vi "trafficlight_main.vi"() -> ()   [LabVIEW 2022 SP3]
panel:
  in  "Stop":bool
  in  "Standby":bool
  out "TrafficLight":cluster{"red":bool, "orange":bool, "green":bool}
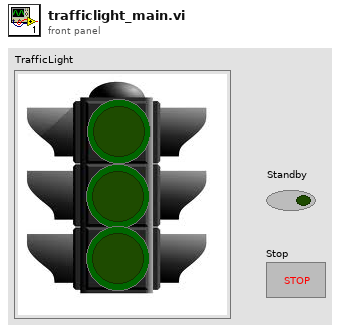
[diagram p1: front panel]
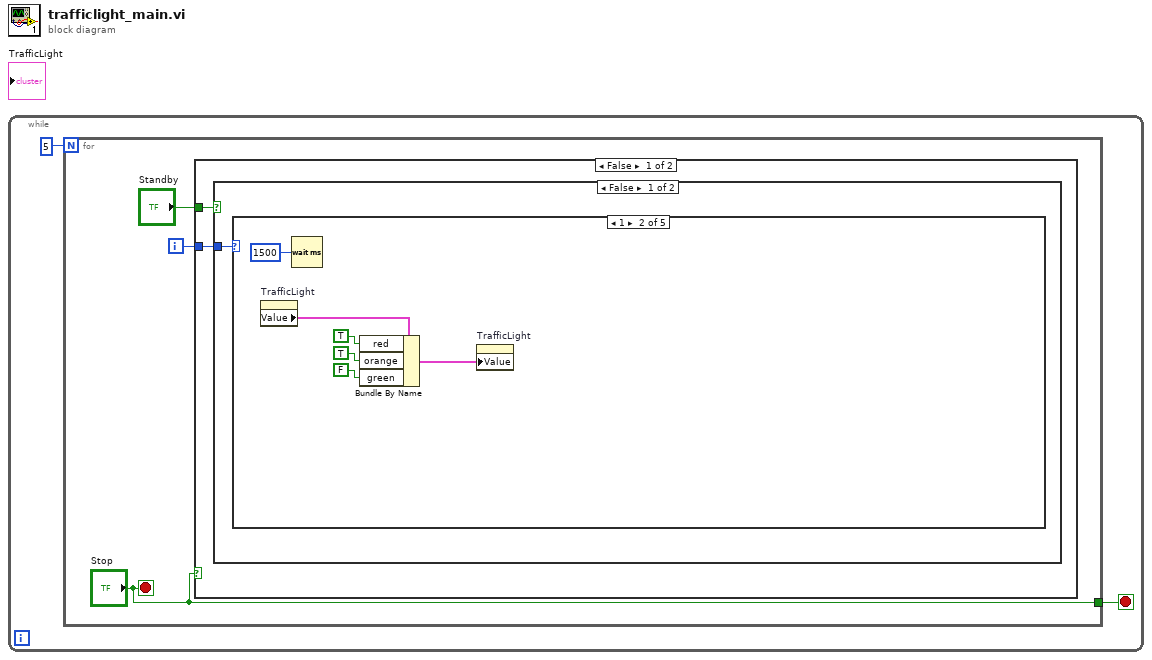
[diagram p0: block diagram]
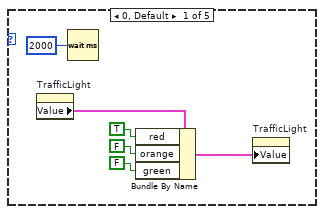
[diagram p2: hidden frame]
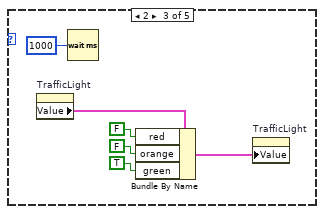
[diagram p3: hidden frame]
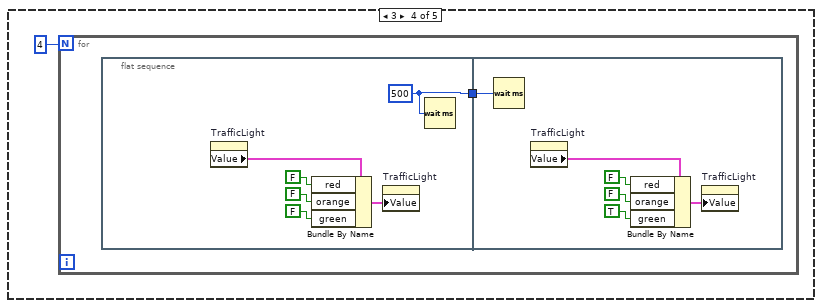
[diagram p4: hidden frame]
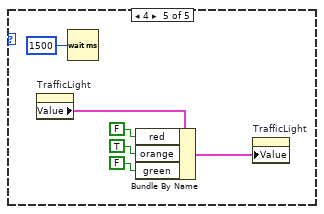
[diagram p5: hidden frame]
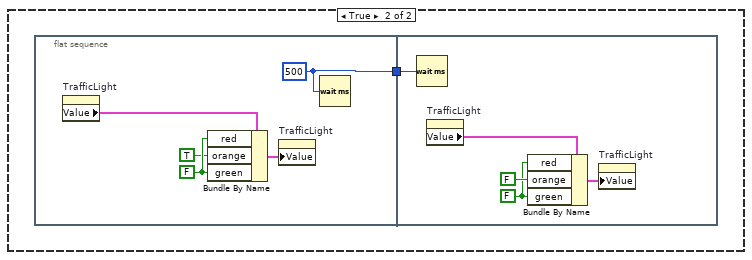
[diagram p6: hidden frame]
diagram:
  n1 = while {
    stop <- w1 stop-if-true
    n2 = for {
      N: 5 -> [_]
      tunnel: ["Stop"] -> w1
      i -> [w5]
      stop <- "Stop" stop-if-true
      n3 = case shown="False" "Stop" {
        tunnel: w5 -> [w7 _]
        tunnel: "Standby" -> [w6 _]
        frame False {
          n4 = case shown="False" w6 {
            tunnel: w7 -> [w8 _]
            frame False {
              n5 = case shown="1" w8 {
                frame 0, Default {
                  n6 = property on="TrafficLight" class="Clust (strict)"() -> ("Value"=w13:cluster{"red":bool, "orange":bool, "green":bool})  [unwired: 2 in, 2 out]
                  n7 = Wait (ms)(milliseconds to wait=u32 2000) -> ()  [unwired: 1 out]
                  n8 = Bundle By Name(cluster=w13, "red"=TRUE, "orange"=FALSE, "green"=FALSE) -> (w12:cluster{"red":bool, "orange":bool, "green":bool})
                  n9 = property on="TrafficLight" class="Clust (strict)"("Value"=w12) -> ()  [unwired: 2 in, 2 out]
                }
                frame 1 {
                  n10 = property on="TrafficLight" class="Clust (strict)"() -> ("Value"=w19:cluster{"red":bool, "orange":bool, "green":bool})  [unwired: 2 in, 2 out]
                  n11 = Wait (ms)(milliseconds to wait=u32 1500) -> ()  [unwired: 1 out]
                  n12 = Bundle By Name(cluster=w19, "red"=TRUE, "orange"=TRUE, "green"=FALSE) -> (w18:cluster{"red":bool, "orange":bool, "green":bool})
                  n13 = property on="TrafficLight" class="Clust (strict)"("Value"=w18) -> ()  [unwired: 2 in, 2 out]
                }
                frame 2 {
                  n14 = property on="TrafficLight" class="Clust (strict)"() -> ("Value"=w25:cluster{"red":bool, "orange":bool, "green":bool})  [unwired: 2 in, 2 out]
                  n15 = Wait (ms)(milliseconds to wait=u32 1000) -> ()  [unwired: 1 out]
                  n16 = Bundle By Name(cluster=w25, "red"=FALSE, "orange"=FALSE, "green"=TRUE) -> (w24:cluster{"red":bool, "orange":bool, "green":bool})
                  n17 = property on="TrafficLight" class="Clust (strict)"("Value"=w24) -> ()  [unwired: 2 in, 2 out]
                }
                frame 3 {
                  n18 = for {
                    N: 4 -> [_]
                    n19 = flat-sequence {
                      tunnel: [w32] -> w28
                      tunnel: w28 -> [w40]
                      frame #0 {
                        w32 = u32 500 ("milliseconds to wait")
                        n20 = property on="TrafficLight" class="Clust (strict)"() -> ("Value"=w34:cluster{"red":bool, "orange":bool, "green":bool})  [unwired: 2 in, 2 out]
                        n21 = Bundle By Name(cluster=w34, "red"=FALSE, "orange"=FALSE, "green"=FALSE) -> (w33:cluster{"red":bool, "orange":bool, "green":bool})
                        n22 = property on="TrafficLight" class="Clust (strict)"("Value"=w33) -> ()  [unwired: 2 in, 2 out]
                        n23 = Wait (ms)(milliseconds to wait=w32) -> ()  [unwired: 1 out]
                      }
                      frame #1 {
                        n24 = Wait (ms)(milliseconds to wait=w40) -> ()  [unwired: 1 out]
                        n25 = property on="TrafficLight" class="Clust (strict)"() -> ("Value"=w38:cluster{"red":bool, "orange":bool, "green":bool})  [unwired: 2 in, 2 out]
                        n26 = Bundle By Name(cluster=w38, "red"=FALSE, "orange"=FALSE, "green"=TRUE) -> (w39:cluster{"red":bool, "orange":bool, "green":bool})
                        n27 = property on="TrafficLight" class="Clust (strict)"("Value"=w39) -> ()  [unwired: 2 in, 2 out]
                      }
                    }
                  }
                }
                frame 4 {
                  n28 = property on="TrafficLight" class="Clust (strict)"() -> ("Value"=w45:cluster{"red":bool, "orange":bool, "green":bool})  [unwired: 2 in, 2 out]
                  n29 = Wait (ms)(milliseconds to wait=u32 1500) -> ()  [unwired: 1 out]
                  n30 = Bundle By Name(cluster=w45, "red"=FALSE, "orange"=TRUE, "green"=FALSE) -> (w44:cluster{"red":bool, "orange":bool, "green":bool})
                  n31 = property on="TrafficLight" class="Clust (strict)"("Value"=w44) -> ()  [unwired: 2 in, 2 out]
                }
              }
            }
            frame True {
              n32 = flat-sequence {
                tunnel: [w48] -> w47
                tunnel: w47 -> [w57]
                frame #0 {
                  w50 = FALSE
                  w48 = u32 500 ("milliseconds to wait")
                  n33 = property on="TrafficLight" class="Clust (strict)"() -> ("Value"=w52:cluster{"red":bool, "orange":bool, "green":bool})  [unwired: 2 in, 2 out]
                  n34 = Bundle By Name(cluster=w52, "red"=w50, "orange"=TRUE, "green"=w50) -> (w51:cluster{"red":bool, "orange":bool, "green":bool})
                  n35 = property on="TrafficLight" class="Clust (strict)"("Value"=w51) -> ()  [unwired: 2 in, 2 out]
                  n36 = Wait (ms)(milliseconds to wait=w48) -> ()  [unwired: 1 out]
                }
                frame #1 {
                  w55 = FALSE
                  n37 = Wait (ms)(milliseconds to wait=w57) -> ()  [unwired: 1 out]
                  n38 = property on="TrafficLight" class="Clust (strict)"() -> ("Value"=w53:cluster{"red":bool, "orange":bool, "green":bool})  [unwired: 2 in, 2 out]
                  n39 = Bundle By Name(cluster=w53, "red"=w55, "orange"=FALSE, "green"=w55) -> (w54:cluster{"red":bool, "orange":bool, "green":bool})
                  n40 = property on="TrafficLight" class="Clust (strict)"("Value"=w54) -> ()  [unwired: 2 in, 2 out]
                }
              }
            }
          }
        }
        frame True {
        }
      }
    }
  }
